vi "Duplicate_AO_WF_4Z.vi"(8 "error in (no error)":errorcluster, 11 "AO WF":waveform(dbl)[](graph)=[{"t0"=timestamp(0 s since 1904-01-01), "dt"=0.0001, "Y"=array[9000 elements]}, {"t0"=timestamp(0 s since 1904-01-01), "dt"=0.0001, "Y"=array[9000 elements]}, {"t0"=timestamp(0 s since 1904-01-01), "dt"=0.0001, "Y"=array[9000 elements]}, {"t0"=timestamp(0 s since 1904-01-01), "dt"=0.0001, "Y"=array[9000 elements]}]) -> (0 "error out":errorcluster, 3 "AO WF 2":waveform(dbl)[](graph))   [LabVIEW 2025]
uses:
  <vilib>/Waveform/WDTOps.llb/WDT Append Waveforms DBL.vi
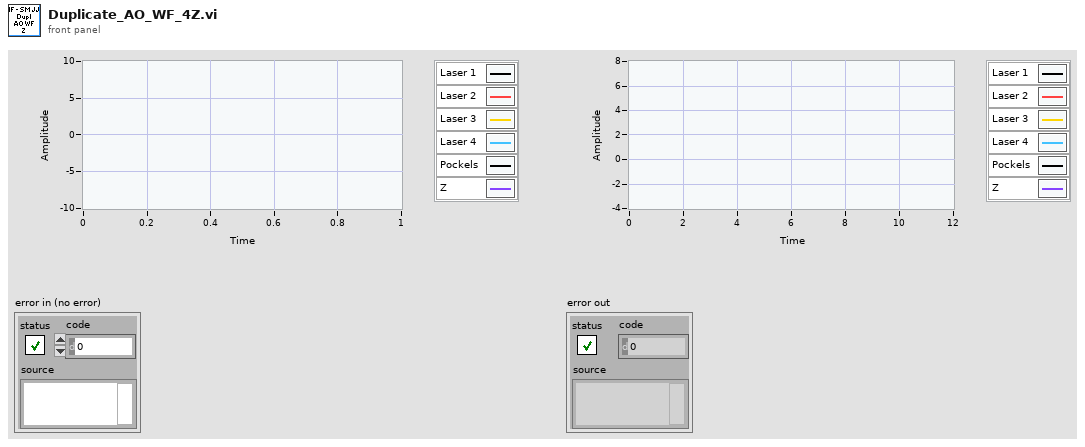
[diagram p1: front panel]
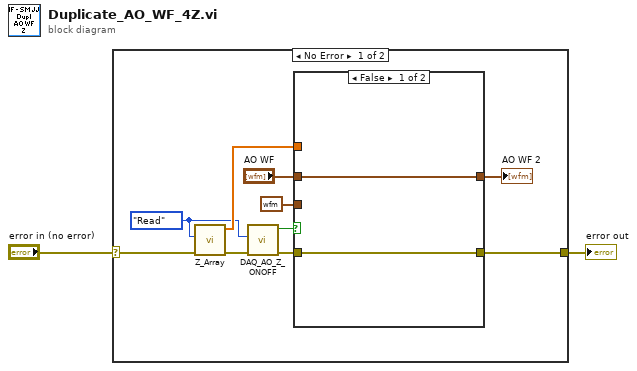
[diagram p0: block diagram]
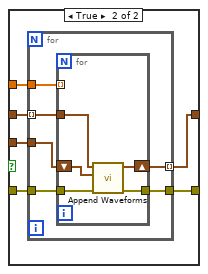
[diagram p2: hidden frame]
diagram:
  n1 = case shown="No Error" "error in (no error)" {
    selector: "error in (no error)" -> [w12 w32]
    tunnel: [w4 w32] -> w2
    frame No Error {
      w7 = enum16{"Init", "Write", "Read"}."Read" ("Action")
      n2 = call "Z_Array.vi"("error in"=w12, "Action"=w7) -> ("error out"=w6:errorcluster, "Z_Array"=w8:dbl[])  [unwired: 8 in]
      n3 = call "DAQ_AO_Z_ONOFF.vi"("error in"=w6, "Action"=w7) -> ("error out"=w5:errorcluster, "ON / OFF"=w3:bool)  [unwired: 8 in]
      n4 = case shown="False" w3 {
        tunnel: "AO WF" -> [w13 w20]
        tunnel: [w13 w19] -> w10
        tunnel: waveform(i32) {"t0"=timestamp(0 s since 1904-01-01), "dt"=1.0, "Y"=[]} ("waveform out") -> [_ w18]
        tunnel: w8 -> [_ w17]
        tunnel: w5 -> [w14 w16]
        tunnel: [w14 w15] -> w4
        frame False {
        }
        frame True {
          n5 = for {
            tunnel: w20 -> [w25] mode=indexing
            tunnel: w18 -> [w26]
            tunnel: [w24] -> w19 mode=indexing
            tunnel: w17 -> [w23]
            tunnel: w16 -> [w22]
            tunnel: [w21] -> w15
            n6 = for {
              tunnel: w25 -> [w30]
              shift-right: [w29] -> w24
              shift-left: w26 -> [w31]
              tunnel: w23 -> [_] mode=indexing
              tunnel: w22 -> [w28]
              tunnel: [w27] -> w21
              n7 = call-poly <vilib>:"Append Waveforms.vi"("error in (no error)"=w28, "waveform B"=w31, "waveform A"=w30) -> ("error out"=w27:errorcluster, "waveform out"=w29:waveform(dbl))  [unwired: 7 in]
            }
          }
        }
      }
      "AO WF 2" <- w10
    }
    frame Error {
    }
  }
  "error out" <- w2
